vi "Show-Attached-Object--Menu-for-BD-Comments.vi"(6 "Mouse Position":T1, 7 "User VI Ref":refnum<vi>, 8 "Is Multi-select?":bool, 9 "Remaining Items":refnum<vi>[](array[refnum]), 10 "Affected Items":T8, 11 "Menu Refnum":refnum<k9>) -> (3 "Menu Items To Add":T2[](array[typedef]))   [LabVIEW 2020]
doc: "This VI is part of a plug-in for modifying the LabVIEW shortcut menus. This is the builder VI which is called when the shortcut menu is built. It tells LabVIEW which shortcut menu items to add to the menu."
uses:
  <resource>/plugins/PopupMenus/support/Checkmark Status.ctl
  <resource>/plugins/PopupMenus/support/Relative Position.ctl
  <resource>/plugins/PopupMenus/support/Position In Menu.ctl
  <resource>/plugins/PopupMenus/support/Transaction Control.ctl
  <resource>/plugins/PopupMenus/support/Shortcut Menu Item Definition.ctl
  <resource>/plugins/PopupMenus/support/Enabled Menu Item Status.ctl
  Show-Attached-Object--Menu-for-BD-Comments.ctl
  <vilib>/Utility/miscctls.llb/LVPositionTypeDef.ctl
panel:
  # "Rules a popup plug-in must follow:\n* This VI's file name must match the file name of the LLB -- only the file extensions should be different.\n* This VI must have debugging disabled or it will be ignored as a plug-in.\n* For all menu items, \"tag suffix + file name of this VI\" must be less than 240 characters.\n* You can disconnect the \"Affected Items\" from the typedef to make the plug-in load faster. The typedef is only there to assist you in keeping this VI and the execution VI using to the same type.\n* All controls on this panel except \"Affected Items\" are locked to prevent accidental edits. Do not change the types or the names of controls other than the elements inside the \"Affected Items\" cluster.\n* See Context Help for more information on the individual controls."
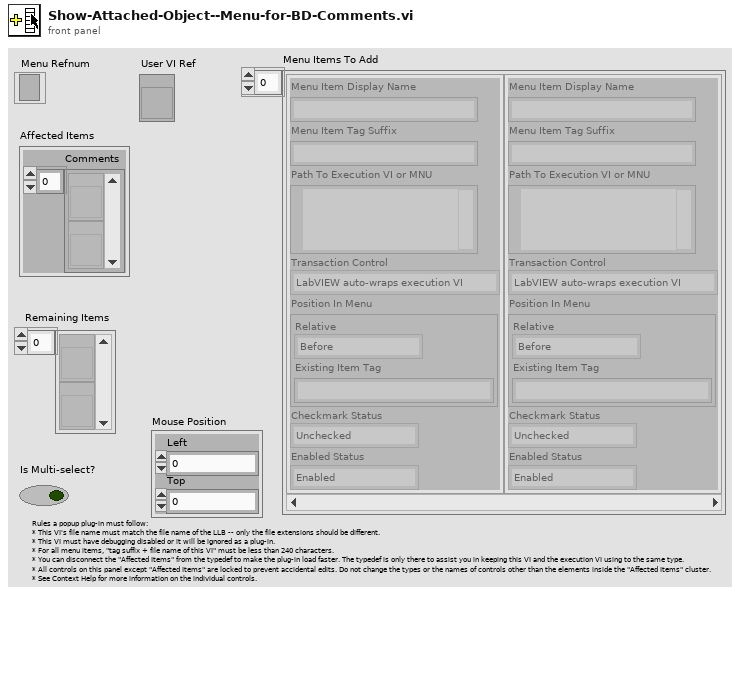
[diagram p1: front panel]
types:
  T1 = typedef "LVPositionTypeDef.ctl" = cluster{"Left":i32, "Top":i32}
  T2 = typedef "Shortcut Menu Item Definition.ctl" = cluster{"Menu Item Display Name":string, "Menu Item Tag Suffix":string, "Path To Execution VI or MNU":path, "Transaction Control":T3, "Position In Menu":T4, "Checkmark Status":T6, "Enabled Status":T7}
  T3 = typedef "Transaction Control.ctl" = enum8{"LabVIEW auto-wraps execution VI", "Execution VI will define if needed"}
  T4 = typedef "Position In Menu.ctl" = cluster{"Relative":T5, "Existing Item Tag":string}
  T5 = typedef "Relative Position.ctl" = enum8{"Before", "Instead of", "After", "Into Submenu"}
  T6 = typedef "Checkmark Status.ctl" = enum8{"Unchecked", "Checked"}
  T7 = typedef "Enabled Menu Item Status.ctl" = enum8{"Enabled", "Disabled"}
  T8 = typedef "Show-Attached-Object--Menu-for-BD-Comments.ctl" = cluster{"Comments":refnum<vi>[]}
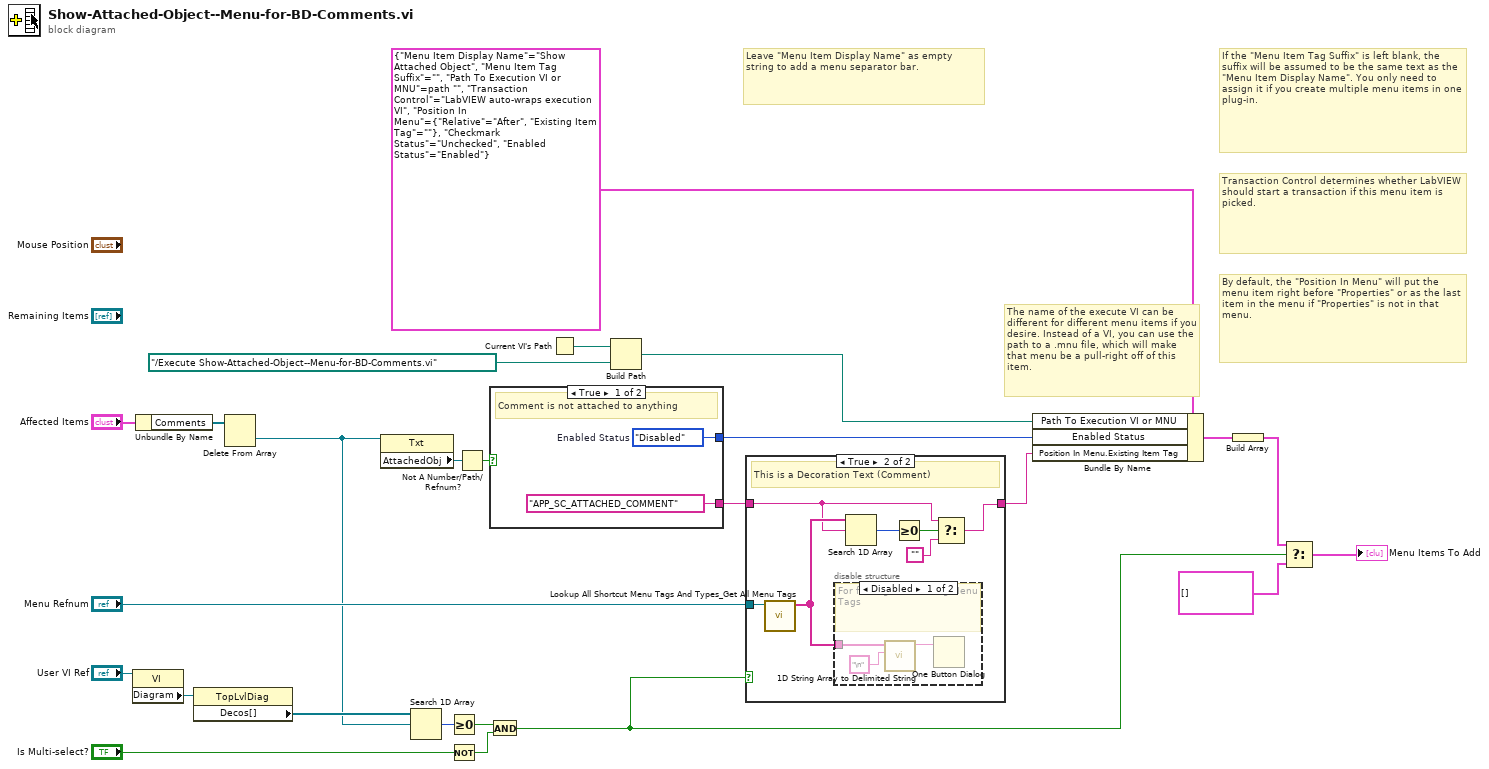
[diagram p0: block diagram]
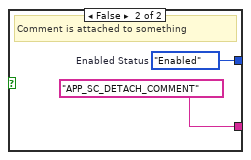
[diagram p4: hidden frame]
diagram:
  # "Transaction Control determines whether LabVIEW should start a transaction if this menu item is picked."
  # "Leave \"Menu Item Display Name\" as empty string to add a menu separator bar."
  # "If the \"Menu Item Tag Suffix\" is left blank, the suffix will be assumed to be the same text as the \"Menu Item Display Name\". You only need to assign it if you create multiple menu items in one plug-in."
  # "By default, the \"Position In Menu\" will put the menu item right before \"Properties\" or as the last item in the menu if \"Properties\" is not in that menu."
  # "The name of the execute VI can be different for different menu items if you desire. Instead of a VI, you can use the path to a .mnu file, which will make that menu be a pull-right off of this item."
  n1 = property class="VI"(reference="User VI Ref") -> ("Diagram"=w6:refnum<vi>)  [unwired: 1 in, 2 out]
  n2 = Unbundle By Name("Affected Items") -> ("Comments"=w19:refnum<vi>[])
  n3 = property class="TopLvlDiag"(reference=w6) -> ("Decos[]"=w5:refnum<vi>[])  [unwired: 1 in, 2 out]
  n4 = Delete From Array(array=w19) -> (deleted portion=w4:refnum<vi>)  [unwired: 2 in, 1 out]
  n5 = property class="Txt"(reference=w4) -> ("AttachedObj"=w18:refnum<vi>)  [unwired: 1 in, 2 out]
  n6 = Search 1D Array(1D array=w5, element=w4) -> (index of element=w12:i32)  [unwired: 1 in]
  n7 = Greater Or Equal To 0?(x=w12) -> (x >= 0?=w9:bool)
  n8 = Not(x="Is Multi-select?") -> (.not. x?=w8:bool)
  n9 = Not A Number/Path/Refnum?(number/path/refnum=w18) -> (NaN/Path/Refnum?=w11:bool)
  n10 = case shown="True" w11 {
    tunnel: [w27 w29] -> w16
    tunnel: ["APP_SC_ATTACHED_COMMENT" ("Position In Menu.Existing Item Tag") "APP_SC_DETACH_COMMENT" ("Position In Menu.Existing Item Tag")] -> w3
    frame True {
      w27 = Enabled_Menu_Item_Status."Disabled"  # Enabled Status
      # "Comment is not attached to anything"
    }
    frame False {
      w29 = Enabled_Menu_Item_Status."Enabled"  # Enabled Status
      # "Comment is attached to something"
    }
  }
  n11 = And(x=w9, y=w8) -> (x .and. y?=w1:bool)
  n12 = Current VI's Path() -> (path=w22:path)
  n13 = Build Path(base path=w22, name or relative path=path "../Execute Show-Attached-Object--Menu-for-BD-Comments.vi" ("execute path")) -> (appended path=w10:path)
  n14 = case shown="True" w1 {
    tunnel: "Menu Refnum" -> [_ w37]
    tunnel: w3 -> [w30 w33]
    tunnel: [w30 w32] -> w2
    frame False {
      # "This is not a Decoration Text (Comment)"
    }
    frame True {
      # "This is a Decoration Text (Comment)"
      n15 = call <resource>:"Lookup All Shortcut Menu Tags And Types_Get All Menu Tags.vi"("menu reference"=w37) -> ("All Menu Tags"=w36:string[])  [unwired: 10 in]
      n16 = disable-structure shown="Disabled" {
        disable-tunnel: w36 -> [w38 _]
        frame Disabled {
          # "For finding the existing Menu Tags"
          n17 = call <vilib>:"1D String Array to Delimited String.vi"("delimiter"="\n", "string array"=w38) -> ("delimited string"=w39:string)  [unwired: 9 in]
          n18 = One Button Dialog(message=w39) -> ()  [unwired: 1 in, 1 out]
        }
        frame Enabled {
        }
      }
      n19 = Search 1D Array(1D array=w36, element=w33) -> (index of element=w35:i32)  [unwired: 1 in]
      n20 = Greater Or Equal To 0?(x=w35) -> (x >= 0?=w34:bool)
      n21 = Select(t=w33, s=w34, f="") -> (s? t:f=w32:string)
    }
  }
  n22 = Bundle By Name(cluster=T2 {"Menu Item Display Name"="Show Attached Object", "Menu Item Tag Suffix"="", "Path To Execution VI or MNU"=path "", "Transaction Control"=enum."LabVIEW auto-wraps execution VI", "Position In Menu"={"Relative"=enum."After", "Existing Item Tag"=""}, "Checkmark Status"=enum."Unchecked", "Enabled Status"=enum."Enabled"} ("Cluster"), "Path To Execution VI or MNU"=w10, "Enabled Status"=w16, "Position In Menu.Existing Item Tag"=w2) -> (w23:T2)
  n23 = Build Array(w23) -> (w15:T2[])
  n24 = Select(t=w15, s=w1, f=T2[] []) -> (s? t:f=→"Menu Items To Add":T2[])
